vi "Set Item.vi"(6 "$Path or Item Name":string, 7 "error in (no error)":errorcluster, 8 "JSON to Insert":string, 9 "Offset":i32, 10 "JSON":string="{}") -> (0 "error out":errorcluster, 1 "Replaced":bool, 3 "<JSON>":string)   [LabVIEW 2017, in "JSONtext.lvlib"]
doc: "Insert or replace JSON item at the $Path specified. Only sets the first found item at the $Path."
uses:
  JSONtext.lvlib
  support/Quote and Escape JSON string.vi
  Parsing/Replace at Offset.vi
  support/Trim Input JSON (and null).vi
  support/quote and escape json string 2.vi
  Parsing/Advance past whitespace.vi
  <vilib>/JDP Science/JDP Science Common Utilities/Trim Whitespace__JDP.vi
  Parsing/Path Notation End Name.vi
  Parsing/Parse Full Path or Item Name.vi
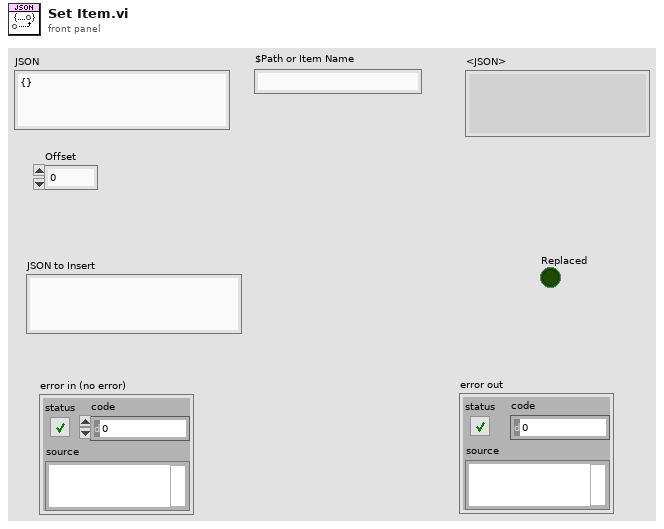
[diagram p1: front panel]
types:
  T1 = typedef "JSONtext.lvlib/Found Items.ctl" = cluster{"Item offset":i32, "Offset past Item":i32, "Name offset":i32, "Offset past Name":i32, "Found":bool, "Item Type":T2, "Item Index":i32}
  T2 = typedef "JSONtext.lvlib/Parsing State.ctl" = enum16{"Parser Error", "Object", "Array", "String", "Number/Other", "Leading Whitespace", "Object end", "Array end", "Value end"}
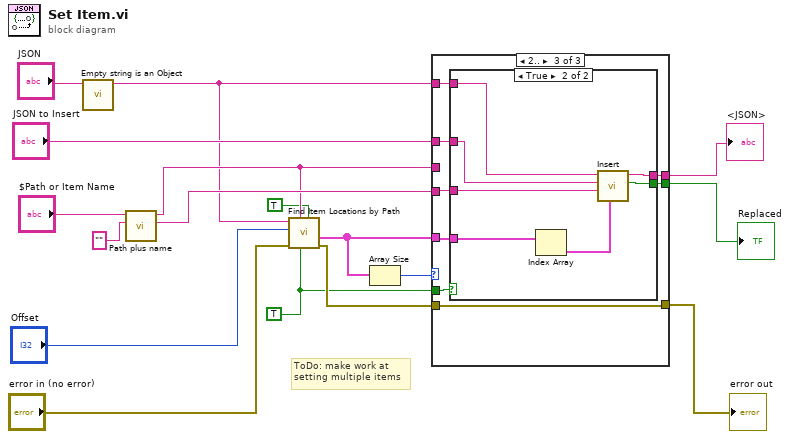
[diagram p0: block diagram]
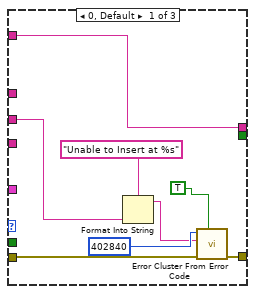
[diagram p2: hidden frame]
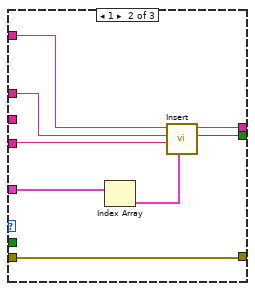
[diagram p3: hidden frame]
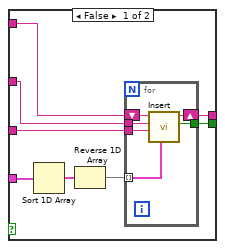
[diagram p4: hidden frame]
diagram:
  w1 = TRUE ("Only return first found")
  # "ToDo: make work at\nsetting multiple items"
  n1 = call "Empty string is an Object.vi"("JSON Input"="JSON") -> ("<JSON>Object"=w7:string)  [unwired: 10 in]
  n2 = call "Path plus name.vi"("Item Name"="", "Object (or Item) Path"="$Path or Item Name") -> ("<JSON>End Name (empty if Array)"=w11:string, "Relative Path or JSON-format name"=w9:string)  [unwired: 7 in, 1 out]
  n3 = call "Find Item Locations by Path.vi"("Insertion point if not found"=TRUE, "Only return first found"=w1, "Path"=w9, "error in (no error)"="error in (no error)", "Offset"="Offset", "JSON"=w7) -> ("error out"=w2:errorcluster, "Items"=w4:T1[])  [unwired: 4 in]
  n4 = Array Size(array=w4) -> (size(s)=w3:i32)
  n5 = case shown="2.." w3 {
    tunnel: "JSON to Insert" -> [_ w33 w41]
    tunnel: [w25 w32 w40] -> w16
    tunnel: w7 -> [w25 w31 w39]
    tunnel: w4 -> [_ w29 w35]
    tunnel: [_ w30 w38] -> w14
    tunnel: w11 -> [_ w27 w37]
    tunnel: w2 -> [w19 w26 w36]
    tunnel: w9 -> [w20 _ _]
    tunnel: [w18 w26 w36] -> w12
    tunnel: w1 -> [_ _ w34]
    frame 0, Default {
      n6 = Format Into String(format string="Unable to Insert at %s", w20) -> (resulting string=w21:string)  [unwired: 2 in, 1 out]
      n7 = call <vilib>:"Error Cluster From Error Code.vi"("show call chain? (False)"=TRUE, "error in (no error)"=w19, "error message (\"\")"=w21, "error code (0)"=402840) -> ("error out"=w18:errorcluster)  [unwired: 5 in]
    }
    frame 1 {
      n8 = Index Array(array=w29) -> (element=w28:T1)  [unwired: 1 in]
      n9 = call "Insert.vi"("Item"=w28, "<JSON>name"=w27, "JSON to Insert"=w33, "JSON in"=w31) -> ("Found"=w30:bool, "string"=w32:string)  [unwired: 5 in, 1 out]
    }
    frame 2.. {
      n10 = case shown="True" w34 {
        tunnel: w41 -> [w49 w57]
        tunnel: [w48 w60] -> w40
        tunnel: w39 -> [w47 w58]
        tunnel: [w46 w61] -> w38
        tunnel: w37 -> [w45 w56]
        tunnel: w35 -> [w44 w59]
        frame False {
          n11 = Sort 1D Array(array=w44) -> (sorted array=w43:T1[])
          n12 = Reverse 1D Array(array=w43) -> (reversed array=w42:T1[])
          n13 = for {
            tunnel: w49 -> [w55]
            tunnel: [w52] -> w46
            tunnel: w45 -> [w51]
            shift-right: [w54] -> w48
            shift-left: w47 -> [w53]
            tunnel: w42 -> [w50] mode=indexing
            n14 = call "Insert.vi"("Item"=w50, "<JSON>name"=w51, "JSON to Insert"=w55, "JSON in"=w53) -> ("Found"=w52:bool, "string"=w54:string)  [unwired: 5 in, 1 out]
          }
        }
        frame True {
          n15 = Index Array(array=w59) -> (element=w62:T1)  [unwired: 1 in]
          n16 = call "Insert.vi"("Item"=w62, "<JSON>name"=w56, "JSON to Insert"=w57, "JSON in"=w58) -> ("Found"=w61:bool, "string"=w60:string)  [unwired: 5 in, 1 out]
        }
      }
    }
  }
  "Replaced" <- w14
  "<JSON>" <- w16
  "error out" <- w12
